vi "Data_to_uart_format.vi"(2 "Payload  Byte to be sent":u8[](array[numeric]), 3 "Type of Message to be sent":T1(ring), 4 "MCU Address to be sent":string(combo)) -> (0 "Byte array has been sent":u8[](array[numeric]), 1 "Converted Message":string)   [LabVIEW 2016]
doc: "The funksjon of this VI is to format you data to a string for the Embedded smart home format.\nThere are 3 inputs and 1 important output. There is also an addition input for view what has been sent.\n\nInput 1: MCU Adress\nInput 2: Message Type\nInput 3: Payload\nOuput 1: String to be sent to UART\n(option) Output 2: Array of the bytes being sent"
panel:
  out "Type of message":T1(ring)
  out "Size of payload":i32
  out "Payload":u8[](array[numeric])
  in  "Intial array":u8[](array[numeric])
  out "MCU address":string
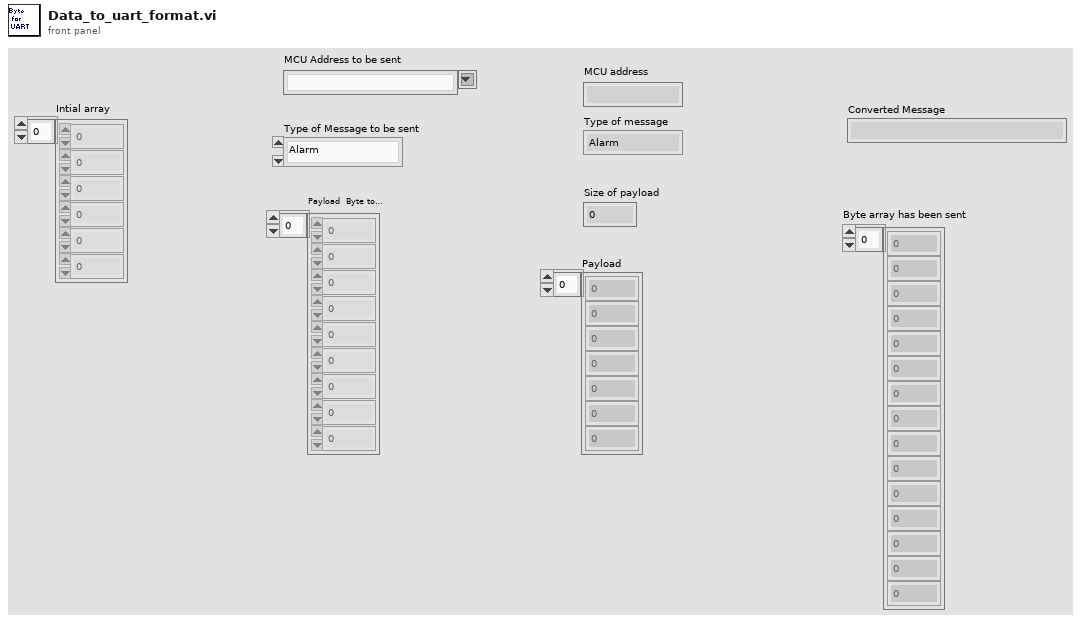
[diagram p1: front panel]
types:
  T1 = enum8{"Alarm", "Error", "Time and date", "Status", "Request"}
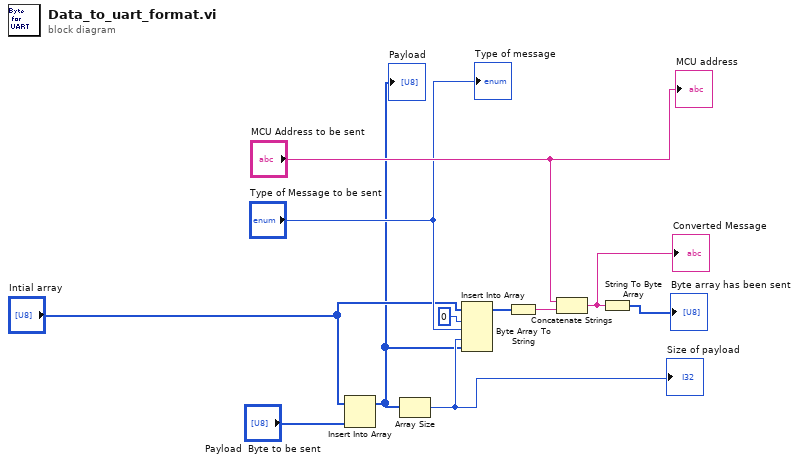
[diagram p0: block diagram]
diagram:
  n1 = Insert Into Array(array="Intial array", new element="Payload  Byte to be sent") -> (w1:u8[])  [unwired: 1 in]
  "Payload" <- w1
  n2 = Array Size(array=w1) -> (size(s)=w7:i32)
  "Size of payload" <- w7
  n3 = Insert Into Array(array="Intial array", index=u8 0, new element #1="Type of Message to be sent", new element #2=w7, new element #3=w1) -> (w8:u8[])
  n4 = Byte Array To String(unsigned byte array=w8) -> (string=w9:string)
  n5 = Concatenate Strings("MCU Address to be sent", w9) -> (w4:string)
  "Converted Message" <- w4
  n6 = String To Byte Array(string=w4) -> (unsigned byte array=→"Byte array has been sent":u8[])
  "MCU address" <- "MCU Address to be sent"
  "Type of message" <- "Type of Message to be sent"
